vi "CANOpen_Main_Prepare status data.vi"(6 "EM timestamp":timestamp, 7 "timestamp":timestamp, 8 "state":u16(ring) items=["unknown"=1, "bootup"=0, "stopped"=4, "operational"=5, "pre-operational"=127, "connection lost"=128], 9 "manufacturer specific error field":u8[](array[numeric]), 10 "EM Error Register":u8, 11 "EM Error Code":u16) -> (3 "element":dbl[](array[numeric]))   [LabVIEW 2013, in "CANOpen Addon Custom Device.lvlib"]
uses:
  CANOpen Addon Custom Device.lvlib
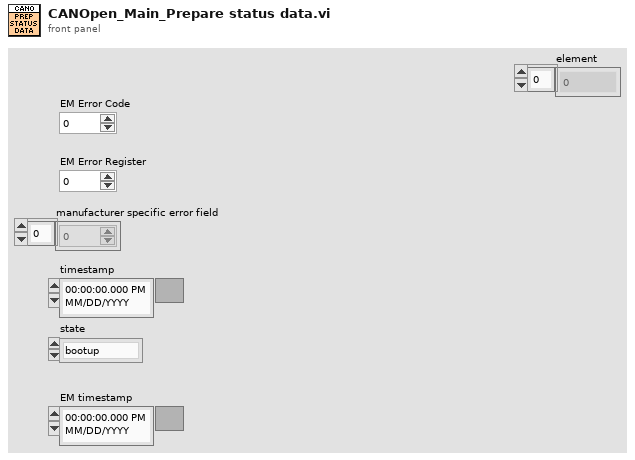
[diagram p1: front panel]
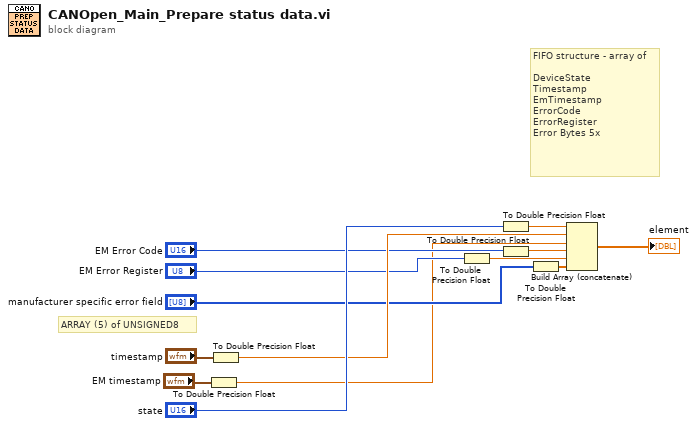
[diagram p0: block diagram]
diagram:
  # "FIFO structure - array of\n\nDeviceState\nTimestamp\nEmTimestamp\nErrorCode\nErrorRegister\nError Bytes 5x"
  # "ARRAY (5) of UNSIGNED8"
  n1 = To Double Precision Float(number="EM timestamp") -> (double precision float=w2:dbl)
  n2 = To Double Precision Float(number="timestamp") -> (double precision float=w10:dbl)
  n3 = To Double Precision Float(number="EM Error Register") -> (double precision float=w7:dbl)
  n4 = To Double Precision Float(number="state") -> (double precision float=w11:dbl)
  n5 = To Double Precision Float(number="EM Error Code") -> (double precision float=w1:dbl)
  n6 = To Double Precision Float(number="manufacturer specific error field") -> (double precision float=w6:dbl[])
  n7 = Build Array (concatenate)(w11, w10, w2, w1, w7, w6) -> (→"element":dbl[])
